vi "Set Crop Mode.vi"(9 "reserved":i32, 10 "cropHeight":i32, 11 "active":i32) -> (3 "function return":u32)   [LabVIEW 2018, in "AndorSDK.lvlib"]
doc: "EXPNETTYPE unsigned int WINAPI SetCropMode(int active, int cropHeight, int reserved);"
uses:
  AndorSDK.lvlib
  ATMCD32D.dll
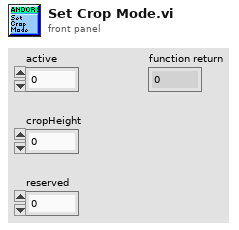
[diagram p1: front panel]
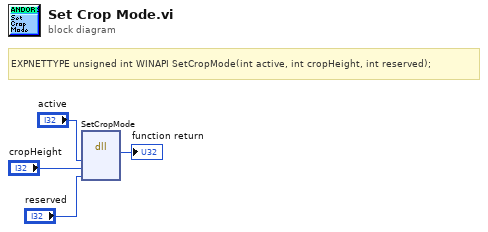
[diagram p0: block diagram]
diagram:
  # "EXPNETTYPE unsigned int WINAPI SetCropMode(int active, int cropHeight, int reserved);"
  n1 = dll-call lib="PTH2babs E\nPersönliches02 - Arbeit03-HiwijobsLabviewCodelibANDOR\tAndor SDK\nATMCD32D.*" fn="SetCropMode"("active"="active", "cropHeight"="cropHeight", "reserved"="reserved") -> (→"function return":u32)  [unwired: 6 in, 2 out]
